vi "Test Execute SQL Query (I64).vi"(8 "error in (no error)":errorcluster, 10 "query":string="SELECT * from employees;", 11 "database in":path=path "C:/labview/sqlite_dbManager/test database/chinook.db") -> (0 "error out":errorcluster, 1 "Query Result":i64[][](array[numeric]), 2 "nonzero result?":bool)   [LabVIEW 2020, in "sqlite3.lvlib"]
uses:
  sqlite3.lvlib
panel:
  in  "desired return type":i64
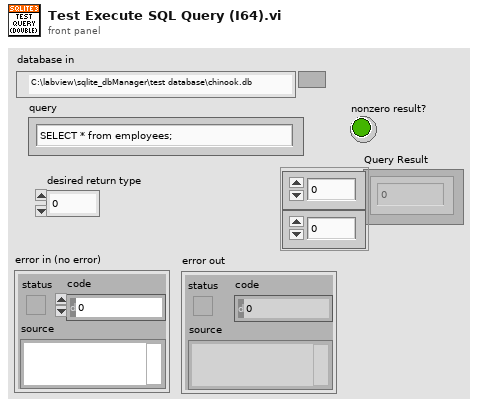
[diagram p1: front panel]
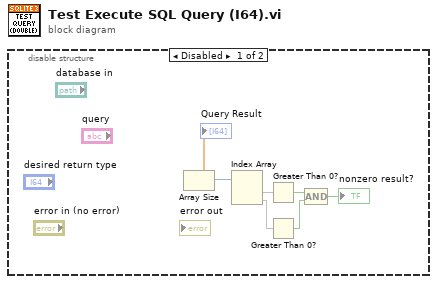
[diagram p0: block diagram]
diagram:
  n1 = disable-structure shown="Disabled" {
    frame Disabled {
      n2 = Array Size() -> (array=→"Query Result":dbl[], size(s)=w6:i32)
      n3 = Index Array(array=w6) -> (element #1=w5, element #2=w4)  [unwired: 2 in]
      n4 = Greater Than 0?(x=w5) -> (x > 0?=w3:bool)
      n5 = Greater Than 0?(x=w4) -> (x > 0?=w2:bool)
      n6 = Compound Arithmetic op=AND(w3, w2) -> (→"nonzero result?":bool)
    }
    frame Enabled {
    }
  }
